vi "CONST ErrorDefinitions.vi"() -> (1 "Error Descriptions":string[](array[string]), 2 "Error Titles":string[](array[string]), 3 "Error Codes":i32[](array[numeric]))   [LabVIEW 2009, in "LD ErrorHandler.lvlib"]
uses:
  LD ErrorHandler.lvlib
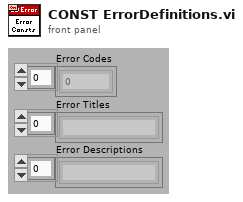
[diagram p1: front panel]
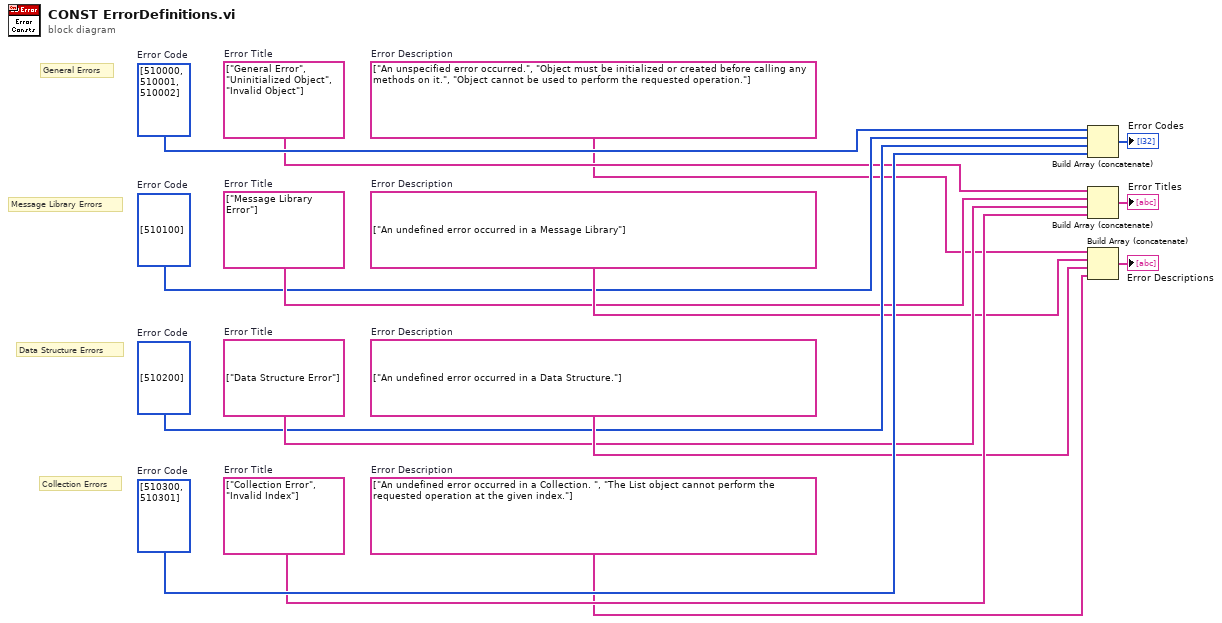
[diagram p0: block diagram]
diagram:
  w9 = string[] ["An undefined error occurred in a Message Library"]  # Error Description
  w7 = i32[] [510100]  # Error Code
  w8 = string[] ["Message Library Error"]  # Error Title
  w12 = string[] ["An undefined error occurred in a Data Structure."]  # Error Description
  w10 = i32[] [510200]  # Error Code
  w11 = string[] ["Data Structure Error"]  # Error Title
  w13 = string[] ["An undefined error occurred in a Collection. ", "The List object cannot perform the requested operation at the given index."]  # Error Description
  w15 = i32[] [510300, 510301]  # Error Code
  w14 = string[] ["Collection Error", "Invalid Index"]  # Error Title
  w4 = string[] ["An unspecified error occurred.", "Object must be initialized or created before calling any methods on it.", "Object cannot be used to perform the requested operation."]  # Error Description
  w6 = i32[] [510000, 510001, 510002]  # Error Code
  w5 = string[] ["General Error", "Uninitialized Object", "Invalid Object"]  # Error Title
  # "Message Library Errors"
  # "Data Structure Errors"
  # "Collection Errors"
  # "General Errors"
  n1 = Build Array (concatenate)(w6, w7, w10, w15) -> (→"Error Codes":i32[])
  n2 = Build Array (concatenate)(w5, w8, w11, w14) -> (→"Error Titles":string[])
  n3 = Build Array (concatenate)(w4, w9, w12, w13) -> (→"Error Descriptions":string[])
